vi "newmark_set_position.vi"(8 "error in":errorcluster, 9 "Axis positions":dbl[](array[numeric]), 11 "VISA Refnum in":refnum<visa-resource-name>) -> (0 "error out":errorcluster, 3 "VISA Refnum out":refnum<visa-resource-name>)   [LabVIEW 2011]
panel:
  # "(degrees)"
  # "Set the controller's position register."
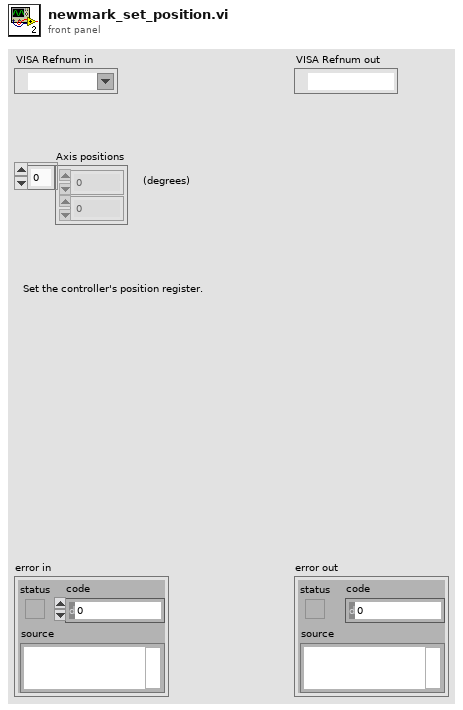
[diagram p1: front panel]
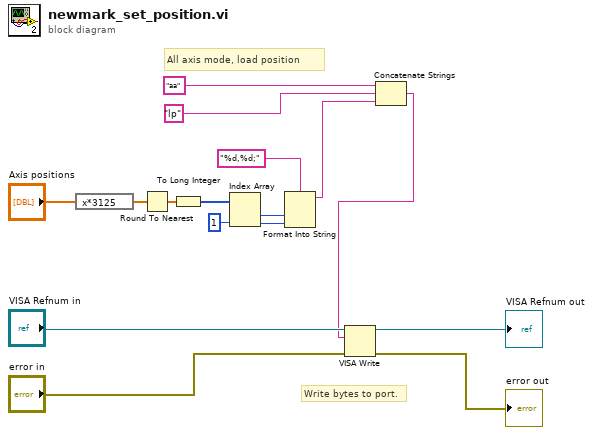
[diagram p0: block diagram]
diagram:
  # "All axis mode, load position"
  # "Write bytes to port."
  n1 = expression code="x*3125"("Axis positions") -> (w12:dbl[])
  n2 = Round To Nearest(number=w12) -> (nearest integer value=w10:dbl[])
  n3 = To Long Integer(number=w10) -> (32bit integer=w9:i32[])
  n4 = Index Array(array=w9, index #2=1 ("index")) -> (element #1=w8:i32, element #2=w7:i32)  [unwired: 1 in]
  n5 = Format Into String(format string="%d,%d;", w8, w7) -> (resulting string=w5:string)  [unwired: 2 in, 1 out]
  n6 = Concatenate Strings("aa" ("string"), "lp" ("string"), w5) -> (w4:string)
  n7 = VISA Write(VISA resource name="VISA Refnum in", write buffer=w4, error in (no error)="error in") -> (VISA resource name out=→"VISA Refnum out":refnum<visa-resource-name>, error out=→"error out":errorcluster)  [unwired: 1 out]
